vi "Configure Measurement.vi"(7 "Scaling (0: Log)":dbl(ring) items=["Log", "Linear"], 8 "error in (no error)":errorcluster, 9 "Combination (0: Single)":dbl(ring) items=["Single", "Feed1-Feed2", "Feed1/Feed2"], 10 "Measurement Number (0: <0>)":i32(ring) items=["Measurement 1"=1, "Measurement 2"=2, "Measurement 3"=3, "Measurement 4"=4], 11 "VISA resource name":refnum<visa-resource-name>) -> (0 "error out":errorcluster, 3 "VISA resource name out":refnum<visa-resource-name>)   [LabVIEW 2011, in "Agilent N432A.lvlib"]
doc: "Configures the measurement mode for the specified window/measurement."
uses:
  <instrlib>/Agilent N432A/Agilent N432A.lvlib
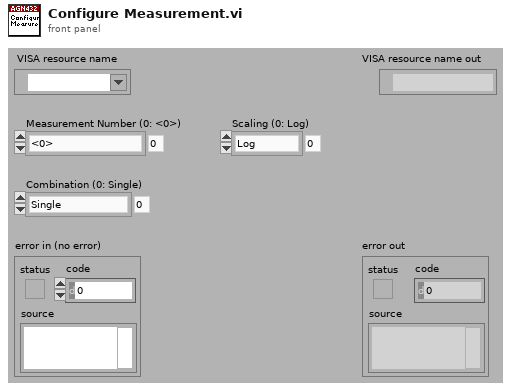
[diagram p1: front panel]
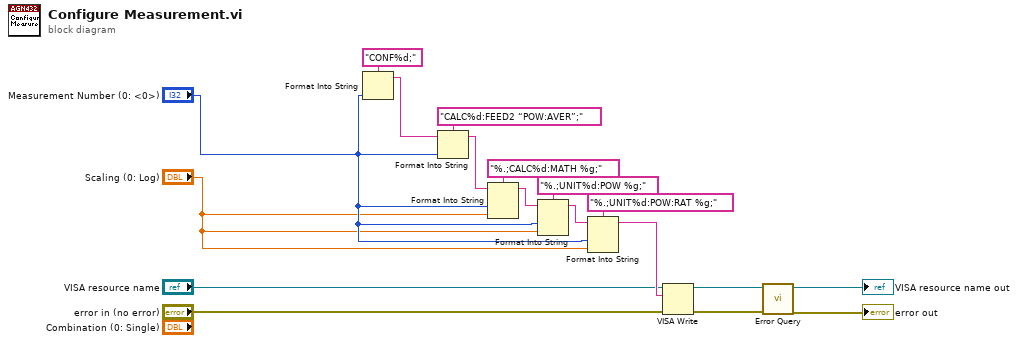
[diagram p0: block diagram]
diagram:
  n1 = Format Into String(format string="CONF%d;", "Measurement Number (0: <0>)") -> (resulting string=w15:string)  [unwired: 2 in, 1 out]
  n2 = Format Into String(format string="CALC%d:FEED2 “POW:AVER”;", initial string=w15, "Measurement Number (0: <0>)") -> (resulting string=w14:string)  [unwired: 1 in, 1 out]
  n3 = Format Into String(format string="%.;CALC%d:MATH %g;", initial string=w14, "Measurement Number (0: <0>)", "Scaling (0: Log)") -> (resulting string=w11:string)  [unwired: 1 in, 1 out]
  n4 = Format Into String(format string="%.;UNIT%d:POW %g;", initial string=w11, "Measurement Number (0: <0>)", "Scaling (0: Log)") -> (resulting string=w9:string)  [unwired: 1 in, 1 out]
  n5 = Format Into String(format string="%.;UNIT%d:POW:RAT %g;", initial string=w9, "Measurement Number (0: <0>)", "Scaling (0: Log)") -> (resulting string=w7:string)  [unwired: 1 in, 1 out]
  n6 = VISA Write(VISA resource name="VISA resource name", write buffer=w7, error in (no error)="error in (no error)") -> (VISA resource name out=w4:refnum<visa-resource-name>, error out=w3:errorcluster)  [unwired: 1 out]
  n7 = call <instrlib>:"Error Query.vi"("error in (no error)"=w3, "VISA resource name"=w4) -> ("error out"=→"error out":errorcluster, "VISA resource name out"=→"VISA resource name out":refnum<visa-resource-name>)  [unwired: 6 in, 2 out]
